vi "Extract Channel Data.vi"(10 "module configuration in":refnum<class "TBM module configuration.lvclass">, 11 "Engine Configuration":refnum<class "engine configuration.lvclass">) -> (1 "Channel Data":string[][](array[string]))   [LabVIEW 2013, in "control module editor.lvclass"]
uses:
  control module editor.lvclass
  <vilib>/NI/Module Execution Interface/Engine Configuration/engine configuration.lvclass
  <vilib>/NI/Tag Bus Module Framework/module configuration/TBM module configuration.lvclass
  <vilib>/NI/Configuration Framework/serializable configuration/NISE_CEF_serializable configuration.lvclass/NISE_CEF_serializable configuration.ctl
  <vilib>/NI/Tag Bus/tag/tag descriptor.lvclass/tag descriptor.ctl
  <vilib>/NI/Tag Bus Module Framework/channel/TBM channel.lvclass/TBM channel.ctl
  <vilib>/Utility/LVClass/Get LV Class Name.vi
  <vilib>/NI/Configuration Framework/error generator.vi
  <vilib>/NI/Tag Bus/tag/tag descriptor.lvclass
  <vilib>/NI/Tag Bus Module Framework/channel/TBM channel.lvclass
  <vilib>/NI/Configuration Framework/serializable configuration/NISE_CEF_serializable configuration.lvclass
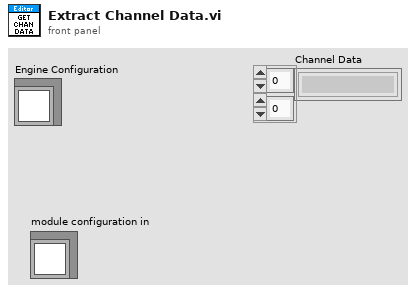
[diagram p1: front panel]
types:
  T1 = typedef "TBM channel.lvclass/channel classification.ctl" = enum16{"input data", "output data", "processing parameter", "processing result"}
  T2 = typedef "tag bus.lvlib/tag descriptor.lvclass/Data Type.ctl" = enum16{"Double", "Single", "I64", "I32", "I16", "I8", "U64", "U32", "U16", "U8", "Boolean", "String", "Array of Double", "Array of Single", "Array of I64", "Array of I32", "Array of I16", "Array of I8", "Array of U64", "Array of U32", "Array of U16", "Array of U8", "Array of Boolean", "Array of String"}
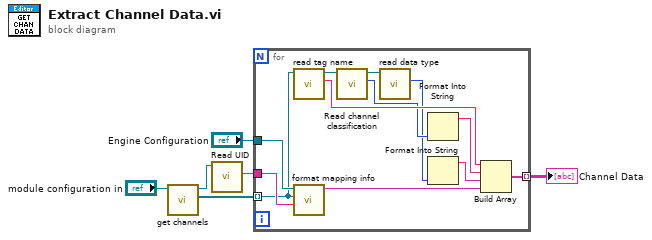
[diagram p0: block diagram]
diagram:
  n1 = call-dynamic "get channels.vi"("module configuration in"="module configuration in") -> ("channels"=w2:refnum<class "TBM channel.lvclass">[], "module configuration out"=w3:refnum<class "TBM module configuration.lvclass">)  [unwired: 9 in]
  n2 = call <vilib>:"Read UID.vi"("configuration in"=w3) -> ("instance id"=w5:string)  [unwired: 8 in, 2 out]
  n3 = for {
    tunnel: w2 -> [w7] mode=indexing
    tunnel: [w17] -> w6 mode=indexing
    tunnel: w5 -> [w16]
    tunnel: "Engine Configuration" -> [w18]
    n4 = call <vilib>:"read tag name.vi"("system tag in"=w7) -> ("name"=w14:string, "system tag out"=w8:refnum<class "TBM channel.lvclass">)  [unwired: 8 in, 1 out]
    n5 = call "format mapping info.vi"("instance id"=w16, "channel"=w7, "engine configuration in"=w18) -> ("mapping info"=w15:string)  [unwired: 8 in]
    n6 = call <vilib>:"Read channel classification.vi"("channel in"=w8) -> ("channel classification"=w13:T1, "channel out"=w10:refnum<class "TBM channel.lvclass">)  [unwired: 8 in, 1 out]
    n7 = call <vilib>:"read data type.vi"("system tag in"=w10) -> ("data type"=w9:T2)  [unwired: 8 in, 2 out]
    n8 = Format Into String(w13) -> (resulting string=w12:string)  [unwired: 3 in, 1 out]
    n9 = Format Into String(w9) -> (resulting string=w11:string)  [unwired: 3 in, 1 out]
    n10 = Build Array(w14, w12, w11, w15) -> (w17:string[])
  }
  "Channel Data" <- w6
